vi "Mousbackground_171213.vi"(11 "input":picture) -> (3 "output-background":picture)   [LabVIEW 2016]
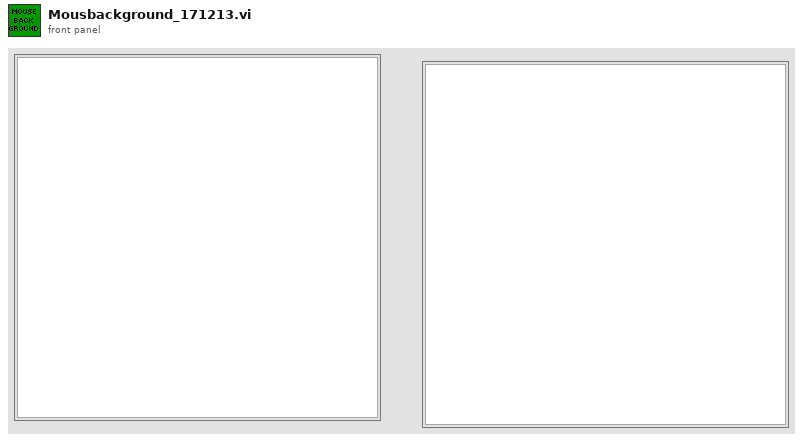
[diagram p1: front panel]
types:
  T1 = cluster{"Width":u16, "Style":enum32{"Solid", "Dash", "Dot", "DashDot", "DashDotDot"}}
  T2 = cluster{"left":i16, "top":i16, "right":i16, "bottom":i16}
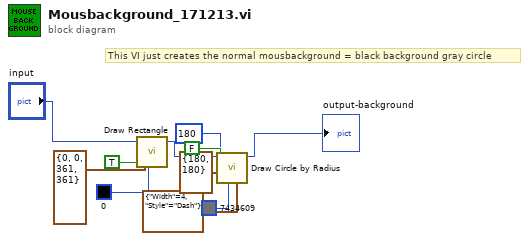
[diagram p0: block diagram]
diagram:
  # "This VI just creates the normal mousbackground = black background gray circle"
  n1 = call <vilib>:"Draw Rectangle.vi"("picture"="input", "rect"=T2 {"left"=0, "top"=0, "right"=361, "bottom"=361}, "fill?(F)"=TRUE, "color(black)"=u32 0) -> ("new picture"=w8:picture)  [unwired: 5 in]
  n2 = call <vilib>:"Draw Circle by Radius.vi"("pen"=T1 {"Width"=4, "Style"=enum."Dash"}, "color(black)"=u32 7434609, "fill?(F)"=FALSE, "pixel center"=cluster{"horizontal":i16, "vertical":i16} {"horizontal"=180, "vertical"=180}, "radius"=i16 180, "picture"=w8) -> ("new picture"=→"output-background":picture)  [unwired: 5 in]
